vi "Solution part 1.vi"() -> ()   [LabVIEW 2020]
uses:
  44e60faa-e688-42fb-b7f1-831ba2913a61.vi
panel:
  out "result":i32
  in  "data?":bool
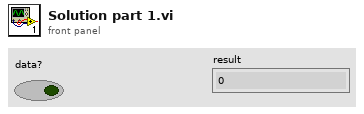
[diagram p1: front panel]
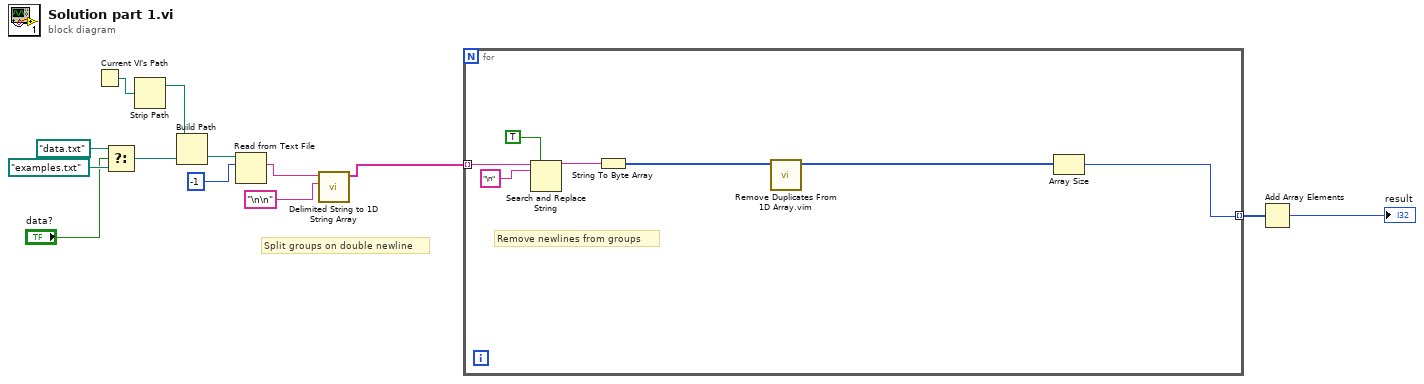
[diagram p0: block diagram]
diagram:
  # "Split groups on double newline"
  n1 = Current VI's Path() -> (path=w9:path)
  n2 = Select(t=path "data.txt", s="data?", f=path "examples.txt") -> (s? t:f=w10:path)
  n3 = Strip Path(path=w9) -> (stripped path=w8:path)  [unwired: 1 out]
  n4 = Build Path(base path=w8, name or relative path=w10) -> (appended path=w7:path)
  n5 = Read from Text File(file (use dialog)=w7, count=-1) -> (text=w4:string)  [unwired: 2 in, 3 out]
  n6 = call <vilib>:"Delimited String to 1D String Array.vi"("delimiter"="\n\n", "delimited string"=w4) -> ("string array"=w3:string[])  [unwired: 9 in]
  n7 = for {
    tunnel: w3 -> [w20] mode=indexing
    tunnel: [w14] -> w1 mode=indexing
    # "Remove newlines from groups"
    n8 = Search and Replace String(replace all?=TRUE ("replace all? (F)"), input string=w20, search string="\n") -> (result string=w17:string)  [unwired: 5 in, 3 out]
    n9 = String To Byte Array(string=w17) -> (unsigned byte array=w16:u8[])
    n10 = call "Remove Duplicates From 1D Array.vim"("array"=w16) -> ("array with duplicates removed"=w15:u8[])  [unwired: 10 in]
    n11 = Array Size(array=w15) -> (size(s)=w14:i32)
  }
  n12 = Add Array Elements(numeric array=w1) -> (sum=→"result":i32)
